vi "Drop Step by Type.vi"(7 "Index":i32, 8 "error in (no error)":errorcluster, 9 "Tag":string, 10 "Step Type Name":string, 11 "SequenceViewPanel in":refnum<class "SequenceViewPanel.lvclass">) -> (0 "error out":errorcluster, 3 "SequenceViewPanel out":refnum<class "SequenceViewPanel.lvclass">)   [LabVIEW 2020, in "TSnax UI.lvlib" / "SequenceViewPanel.lvclass"]
uses:
  SequenceViewPanel.lvclass
  TSnax/TS License Type.ctl
  SequenceViewPanel.lvclass/SequenceViewPanel.ctl
  TSnax/SequenceFile/SequenceFile.lvclass
  TSnax/Engine/Engine.lvclass
  TSnax/TSnax.lvlib
  TSnax/Step/Step.lvclass
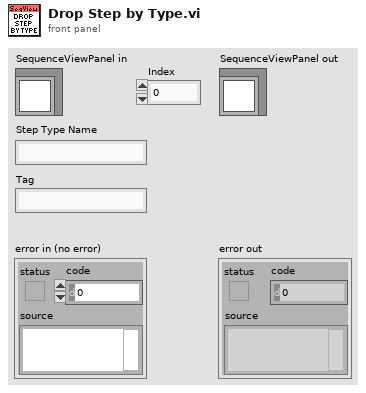
[diagram p1: front panel]
types:
  T1 = typedef "TSnax.lvlib/TS License Type.ctl" = enum16{"Operator", "CustomEditor", "SequenceEditor"}
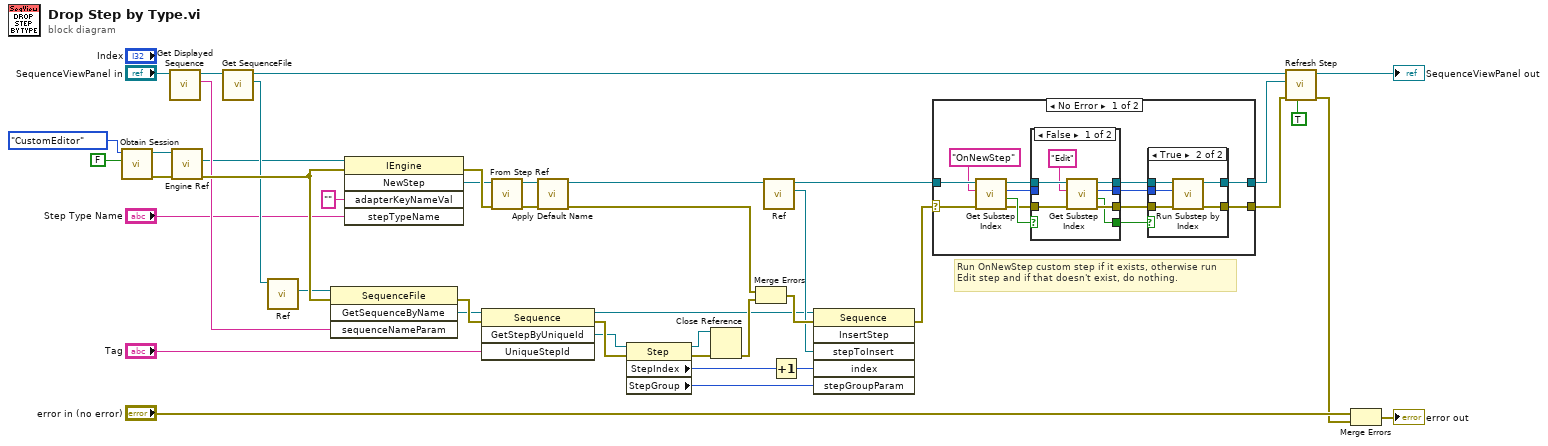
[diagram p0: block diagram]
diagram:
  # "Run OnNewStep custom step if it exists, otherwise run Edit step and if that doesn't exist, do nothing."
  n1 = call "Obtain Session.vi"("Create if needed? (T)"=FALSE, "TS License Type (Operator)"=TS_License_Type."CustomEditor") -> ("error out"=w32:errorcluster, "Engine out"=w33:refnum<class "Engine.lvclass">)  [unwired: 8 in]
  n2 = call "Get Displayed Sequence.vi"("SequenceViewPanel in"="SequenceViewPanel in") -> ("Sequence"=w34:string, "SequenceViewPanel out"=w37:refnum<class "SequenceViewPanel.lvclass">)  [unwired: 8 in, 1 out]
  n3 = call "Engine Ref.vi"("error in (no error)"=w32, "Engine in"=w33) -> ("error out"=w40:errorcluster, "Engine"=w29:refnum<k7>)  [unwired: 7 in, 1 out]
  n4 = call "Get SequenceFile.vi"("SequenceViewPanel in"=w37) -> ("SequenceFile"=w36:refnum<class "SequenceFile.lvclass">, "SequenceViewPanel out"=w1:refnum<class "SequenceViewPanel.lvclass">)  [unwired: 8 in, 1 out]
  n5 = call "Ref.vi"("SequenceFile in"=w36) -> ("Ref"=w35:refnum<k7>)  [unwired: 8 in, 2 out]
  n6 = invoke class="SequenceFile" method="GetSequenceByName"(reference=w35, error in=w40, "sequenceNameParam"=w34) -> (error out=w42:errorcluster, "GetSequenceByName"=w14:refnum<k7>)  [unwired: 1 in, 2 out]
  n7 = invoke class="IEngine" method="NewStep"(reference=w29, error in=w40, "adapterKeyNameVal"="", "stepTypeName"="Step Type Name") -> (error out=w41:errorcluster, "NewStep"=w26:refnum<k7>)  [unwired: 1 in, 3 out]
  n8 = invoke class="Sequence" method="GetStepByUniqueId"(reference=w14, error in=w42, "UniqueStepId"="Tag") -> (reference out=w3:refnum<k7>, error out=w43:errorcluster, "GetStepByUniqueId"=w12:refnum<k7>)  [unwired: 1 in, 1 out]
  n9 = call "From Step Ref.vi"("error in (no error)"=w41, "Ref"=w26) -> ("error out"=w15:errorcluster, "Step out"=w16:refnum<class "Step.lvclass">)  [unwired: 8 in]
  n10 = call "Apply Default Name.vi"("error in (no error)"=w15, "Step in"=w16) -> ("error out"=w9:errorcluster, "Step out"=w2:refnum<class "Step.lvclass">)  [unwired: 8 in]
  n11 = property class="Step"(reference=w12, error in=w43) -> (reference out=w7:refnum<k7>, error out=w8:errorcluster, "StepIndex"=w10:i32, "StepGroup"=w11:i32)
  n12 = Close Reference(reference=w7, error in (no error)=w8) -> (error out=w6:errorcluster)
  n13 = Merge Errors(w9, w6) -> (w5:errorcluster)
  n14 = call "Ref.vi"("Step in"=w2) -> ("Step"=w4:refnum<k7>, "Step out"=w23:refnum<class "Step.lvclass">)  [unwired: 8 in, 1 out]
  n15 = Increment(x=w10) -> (x+1=w25:i32)
  n16 = invoke class="Sequence" method="InsertStep"(reference=w3, error in=w5, "stepToInsert"=w4, "index"=w25, "stepGroupParam"=w11) -> (error out=w22:errorcluster)  [unwired: 1 in, 5 out]
  n17 = case shown="No Error" w22 {
    selector: w22 -> [w55 w75]
    tunnel: w23 -> [w56 w76]
    tunnel: [w46 w76] -> w21
    tunnel: [w45 w75] -> w19
    frame No Error {
      n18 = call "Get Substep Index.vi"("error in (no error)"=w55, "Substep Name"="OnNewStep", "Step in"=w56) -> ("error out"=w52:errorcluster, "Has Named Substep?"=w53:bool, "Index"=w50:i32, "Step out"=w51:refnum<class "Step.lvclass">)  [unwired: 5 in]
      n19 = case shown="False" w53 {
        selector: w53 -> [_ w71]
        tunnel: w52 -> [w69 w72]
        tunnel: w51 -> [w70 w73]
        tunnel: w50 -> [_ w74]
        tunnel: [w67 w72] -> w48
        tunnel: [w66 w73] -> w49
        tunnel: [w65 w74] -> w47
        tunnel: [w64 w71] -> w44
        frame False {
          n20 = call "Get Substep Index.vi"("error in (no error)"=w69, "Substep Name"="Edit", "Step in"=w70) -> ("error out"=w67:errorcluster, "Has Named Substep?"=w64:bool, "Index"=w65:i32, "Step out"=w66:refnum<class "Step.lvclass">)  [unwired: 5 in]
        }
        frame True {
        }
      }
      n21 = case shown="True" w44 {
        tunnel: w49 -> [w58 w63]
        tunnel: w48 -> [w57 w62]
        tunnel: w47 -> [_ w61]
        tunnel: [w58 w60] -> w46
        tunnel: [w57 w59] -> w45
        frame False {
        }
        frame True {
          n22 = call "Run Substep by Index.vi"("error in (no error)"=w62, "Substep Index"=w61, "Step in"=w63) -> ("error out"=w59:errorcluster, "Step out"=w60:refnum<class "Step.lvclass">)  [unwired: 6 in, 1 out]
        }
      }
    }
    frame Error {
    }
  }
  n23 = call "Refresh Step.vi"("Skip Response? (F)"=TRUE, "error in (no error)"=w19, "Step"=w21, "SequenceViewPanel in"=w1) -> ("error out"=w18:errorcluster, "SequenceViewPanel out"=→"SequenceViewPanel out":refnum<class "SequenceViewPanel.lvclass">)  [unwired: 6 in]
  n24 = Merge Errors("error in (no error)", w18) -> (→"error out":errorcluster)
